vi "Insert Panel.vi"(5 "Display Type":refnum<class "ArrayPanel.lvclass">, 8 "error in (no error)":errorcluster, 9 "Position (End)":i32=-1, 10 "Panel/Type":refnum<class "ArrayPanel.lvclass">, 11 "PanelArray in":refnum<class "ArrayManager.lvclass">) -> (0 "error out":errorcluster, 2 "Panel":refnum<class "ArrayPanel.lvclass">, 3 "PanelArray out":refnum<class "ArrayManager.lvclass">)   [LabVIEW 2020, in "OOPanel.lvlib" / "ArrayManager.lvclass"]
uses:
  ArrayManager.lvclass
  ArrayPanel/ArrayPanel.lvclass
  C:/dev/LabVIEW/lv-oopanel/OOPanel/Panel/Panel.lvclass
  Panel/Panel.lvclass/Panel.ctl
  ArrayManager.lvclass/ArrayManager.ctl
  ArrayPanel/ArrayPanel.lvclass/ArrayPanel.ctl
  <vilib>/Utility/error.llb/Error Cluster From Error Code.vi
  <vilib>/ErrorRing/Error Ring.xnode
  Panel/Panel.lvclass
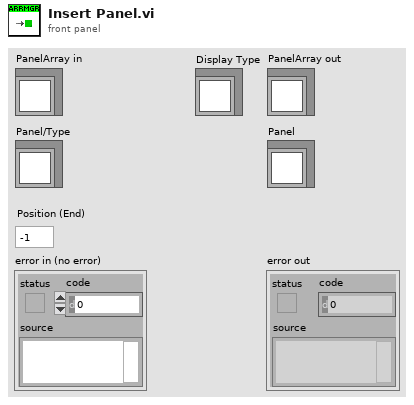
[diagram p1: front panel]
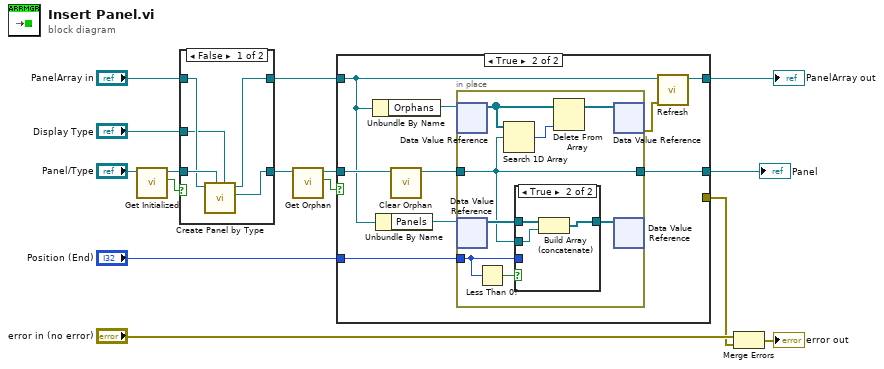
[diagram p0: block diagram]
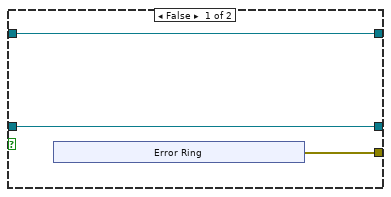
[diagram p3: hidden frame]
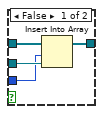
[diagram p4: hidden frame]
diagram:
  n1 = call "Get Initialized.vi"("Panel in"="Panel/Type") -> ("Initialized"=w7:bool, "Panel out"=w6:refnum<class "ArrayPanel.lvclass">)  [unwired: 8 in, 1 out]
  n2 = case shown="False" w7 {
    tunnel: w6 -> [w20 w22]
    tunnel: [w17 w22] -> w5
    tunnel: "PanelArray in" -> [w19 w21]
    tunnel: [w18 w21] -> w3
    tunnel: "Display Type" -> [w16 _]
    frame False {
      n3 = call "Create Panel by Type.vi"("Display Type"=w16, "Panel Type"=w20, "PanelArray in"=w19) -> ("Panel"=w17:refnum<class "ArrayPanel.lvclass">, "PanelArray out"=w18:refnum<class "ArrayManager.lvclass">)  [unwired: 6 in, 1 out]
    }
    frame True {
    }
  }
  n4 = call "Get Orphan.vi"("ArrayPanel in"=w5) -> ("Orphan"=w14:bool, "ArrayPanel out"=w13:refnum<class "ArrayPanel.lvclass">)  [unwired: 8 in, 1 out]
  n5 = case shown="True" w14 {
    tunnel: w3 -> [w24 w32]
    tunnel: w13 -> [w23 w37]
    tunnel: [w25 _] -> w10
    tunnel: "Position (End)" -> [_ w35]
    tunnel: [w24 w33] -> w9
    tunnel: [w23 w30] -> w2
    frame False {
      n6 = xnode "Error Ring"() -> ("error out"=w25:errorcluster)
    }
    frame True {
      n7 = Unbundle By Name(w32) -> ("Orphans"=w38:refnum<data-value>)
      n8 = Unbundle By Name(w32) -> ("Panels"=w36:refnum<data-value>)
      n9 = call "Clear Orphan.vi"("ArrayPanel in"=w37) -> ("ArrayPanel out"=w31:refnum<class "ArrayPanel.lvclass">)  [unwired: 9 in, 1 out]
      n10 = in-place {
        in-place-border: w31 -> [w39]
        in-place-border: w35 -> [w41]
        in-place-border: [w39] -> w30
        n11 = in-place-dvr #1(w38) -> (w46:refnum<class "ArrayPanel.lvclass">[])  [unwired: 1 out]
        n12 = in-place-dvr #2(w36) -> (w43:refnum<class "ArrayPanel.lvclass">[])  [unwired: 1 out]
        n13 = Less Than 0?(x=w41) -> (x < 0?=w40:bool)
        n14 = Search 1D Array(1D array=w46, element=w39) -> (index of element=w44:i32)  [unwired: 1 in]
        n15 = case shown="True" w40 {
          tunnel: w41 -> [w48 _]
          tunnel: w43 -> [w50 w53]
          tunnel: w39 -> [w49 w52]
          tunnel: [w47 w51] -> w42
          frame False {
            n16 = Insert Into Array(array=w50, index=w48, new element=w49) -> (w47:refnum<class "ArrayPanel.lvclass">[])
          }
          frame True {
            n17 = Build Array (concatenate)(w53, w52) -> (w51:refnum<class "ArrayPanel.lvclass">[])
          }
        }
        n18 = Delete From Array(array=w46, index=w44) -> (array with subset deleted=w45:refnum<class "ArrayPanel.lvclass">[])  [unwired: 1 in, 1 out]
        n19 = in-place-dvr #1(w45) -> (w34:errorcluster)  [unwired: 1 out]
        n20 = in-place-dvr #2(w42) -> ()  [unwired: 2 out]
      }
      n21 = call "Refresh.vi"("error in (no error)"=w34, "ArrayManager in"=w32) -> ("ArrayManager out"=w33:refnum<class "ArrayManager.lvclass">)  [unwired: 8 in, 1 out]
    }
  }
  "PanelArray out" <- w9
  "Panel" <- w2
  n22 = Merge Errors("error in (no error)", w10) -> (→"error out":errorcluster)
